vi "getElfByIndex.vi"(8 "error in (no error)":errorcluster, 10 "Index":i32, 11 "ElfHeap in":refnum<class "ElfHeap.lvclass">) -> (0 "error out":errorcluster, 2 "Elf":refnum<class "Elf.lvclass">)   [LabVIEW 2017, in "ElfHeap.lvclass"]
uses:
  ElfHeap.lvclass
  Elf/Elf.lvclass
  ElfHeap.lvclass/ElfHeap.ctl
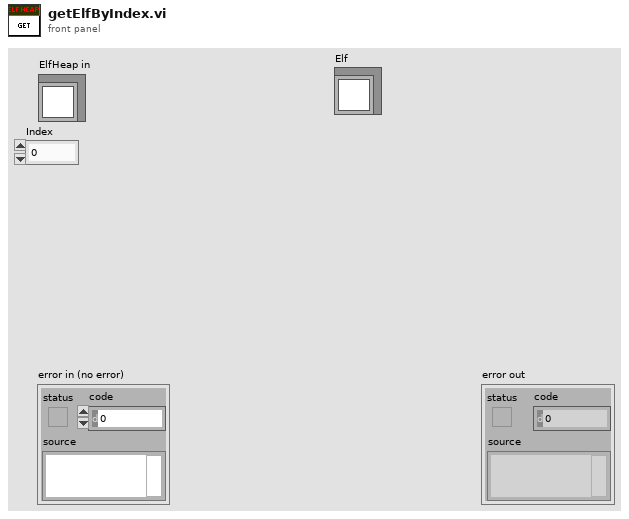
[diagram p1: front panel]
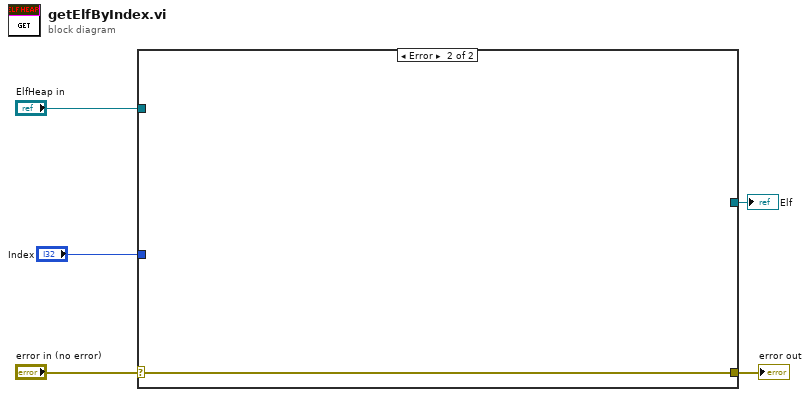
[diagram p0: block diagram]
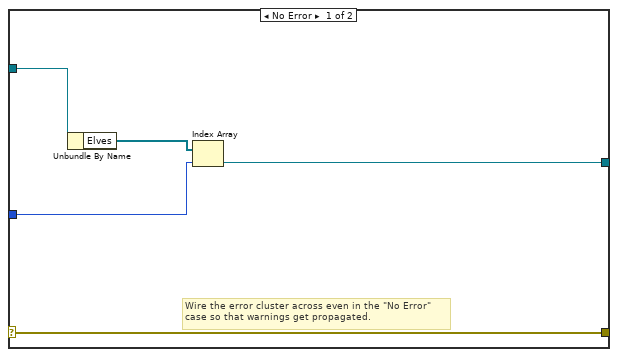
[diagram p2: hidden frame]
diagram:
  n1 = case shown="Error" "error in (no error)" {
    selector: "error in (no error)" -> [w10 w11]
    tunnel: [w10 w11] -> w4
    tunnel: "ElfHeap in" -> [w9 _]
    tunnel: "Index" -> [w7 _]
    tunnel: [w6 _] -> w1
    frame No Error {
      # "Wire the error cluster across even in the \"No Error\"\ncase so that warnings get propagated."
      n2 = Unbundle By Name(w9) -> ("Elves"=w8:refnum<class "Elf.lvclass">[])
      n3 = Index Array(array=w8, index=w7) -> (element=w6:refnum<class "Elf.lvclass">)
    }
    frame Error {
    }
  }
  "error out" <- w4
  "Elf" <- w1
